vi "Arduino_data.vi"() -> ()   [LabVIEW 2017]
panel:
  out "Waveform Chart":waveform(i32)(graph)
  in  "stop":bool
  in  "Samples qty":i32
  in  "Period (ms)":u32=10
  in  "COM Port":refnum<visa-resource-name>="COM1"
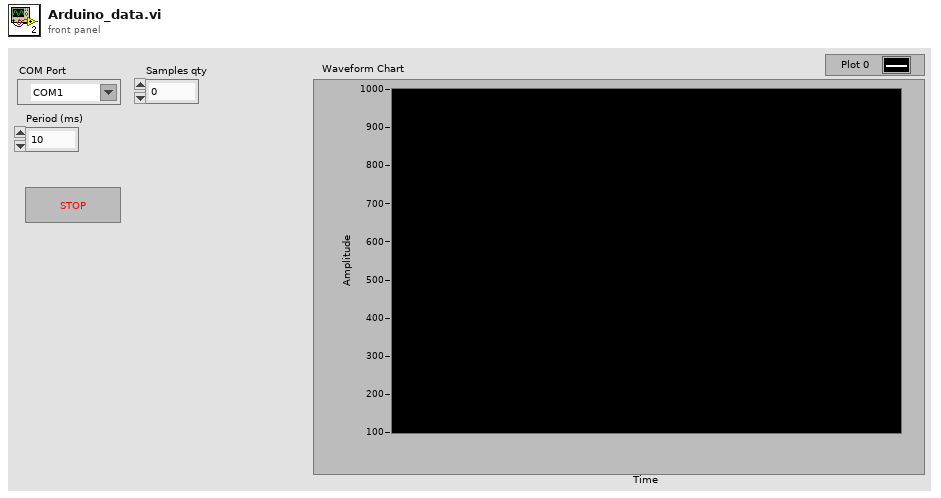
[diagram p1: front panel]
types:
  T1 = typedef "device.ctl" = cluster{"Device Session":refnum<visa-resource-name>, "dT":i32}
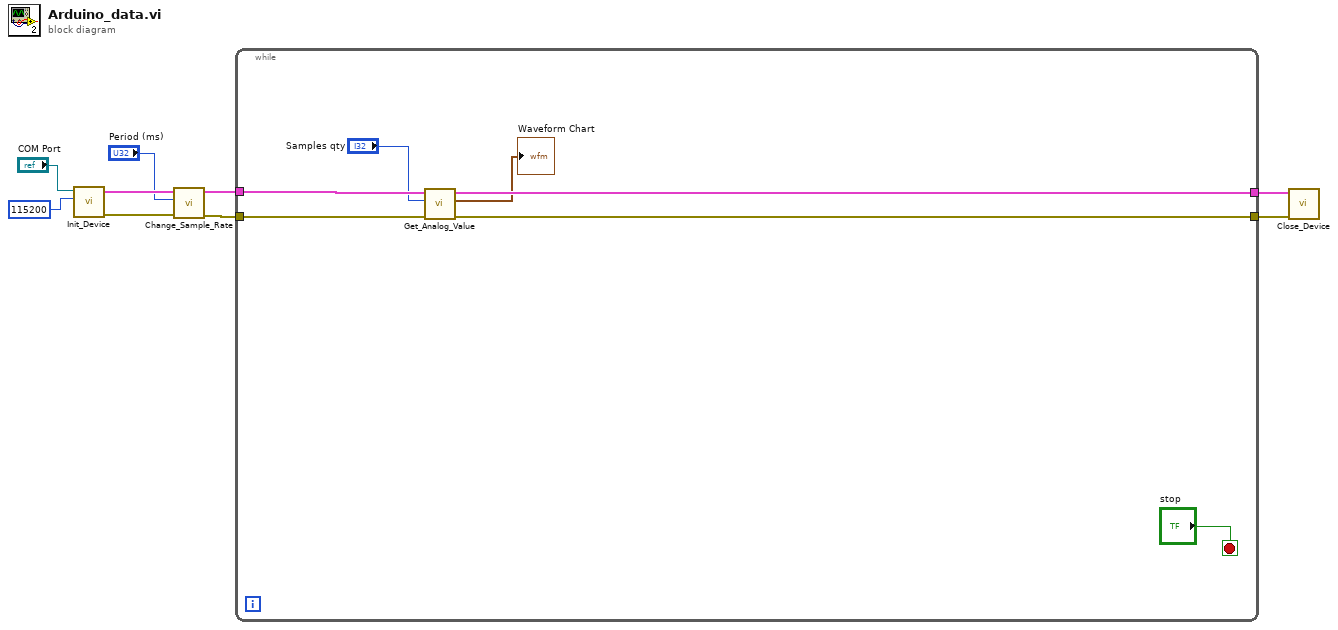
[diagram p0: block diagram]
diagram:
  n1 = call "Init_Device.vi"("Baud Rate (115200)"=u32 115200 ("Baud Rate"), "COM Port"="COM Port") -> ("error out"=w6:errorcluster, "Device"=w7:T1)  [unwired: 8 in]
  n2 = call "Change_Sample_Rate.vi"("error in"=w6, "Period [ms]"="Period (ms)", "Device IN"=w7) -> ("error out"=w5:errorcluster, "Device OUT"=w4:T1)  [unwired: 7 in]
  n3 = while {
    tunnel: w5 -> [w16]
    tunnel: w4 -> [w15]
    tunnel: [w12] -> w3
    tunnel: [w11] -> w1
    stop <- "stop" stop-if-true
    n4 = call "Get_Analog_Value.vi"("error in"=w16, "Samples qty (1)"="Samples qty", "Device IN"=w15) -> ("error out"=w12:errorcluster, "output waveform"=→"Waveform Chart":waveform(i32), "Device OUT"=w11:T1)  [unwired: 5 in]
  }
  n5 = call "Close_Device.vi"("error in"=w3, "Device IN"=w1) -> ()  [unwired: 8 in, 1 out]
